vi "WPI_MotorControlSetOutput.vi"(8 "error in (no error)":errorcluster, 9 "options":u8, 10 "Output":dbl, 11 "MotorControlDevRef":T1={"DeviceStatus"={"status"=FALSE, "code"=0, "source"=""}, "Type"=enum."PWM", "PWM"={"PWM Channel"=enum."Invalid", "DeadBand"={"Name"="", "maxPositivePwm"=0, "minPositivePwm"=0, "centerPwm"=0, "maxNegativePwm"=0, "minNegativePwm"=0, "angularRange"=0}}, "CAN"={"Device Number"=0, "SetOutput VI Ref"=variant(refnum<vi> refnum), "GetOutput VI Ref"=variant(refnum<vi> refnum), "Enable VI Ref"=variant(refnum<vi> refnum), "Disable VI Ref"=variant(refnum<vi> refnum), "Data"=variant}, "Invert"=FALSE, "DIO PWM"={"PWM \"Enable\" Channel"=enum."Invalid", "DIOChannel"=enum."Invalid", "PWM Rate"=0.0}}) -> (0 "error out":errorcluster, 2 "Motor Output":dbl, 3 "MotorControlDevRef":T1={"DeviceStatus"={"status"=FALSE, "code"=0, "source"=""}, "Type"=enum."PWM", "PWM"={"PWM Channel"=enum."Invalid", "DeadBand"={"Name"="", "maxPositivePwm"=0, "minPositivePwm"=0, "centerPwm"=0, "maxNegativePwm"=0, "minNegativePwm"=0, "angularRange"=0}}, "CAN"={"Device Number"=0, "SetOutput VI Ref"=variant(refnum<vi> refnum), "GetOutput VI Ref"=variant(refnum<vi> refnum), "Enable VI Ref"=variant(refnum<vi> refnum), "Disable VI Ref"=variant(refnum<vi> refnum), "Data"=variant}, "Invert"=FALSE, "DIO PWM"={"PWM \"Enable\" Channel"=enum."Invalid", "DIOChannel"=enum."Invalid", "PWM Rate"=0.0}})   [LabVIEW 2025]
doc: "Specifies the output value or set-point for the motor controller.\n\nIf you use a motor controller connected to PWM, the scaled value can range from -1.0 to 1.0.\n\nIf you use a CAN Jaguar, the scale and the units depend on the mode the Jaguar is in. In <B>Percent VBus</B> mode, the range is the same as the PWM interface. In <B>Voltage</B>, <B>Current</B>, <B>Speed</B>, and <B>Position</B> modes, the <B>Output</B> is specified in engineering units (Volts, Amps, Rotations/Minute, and Rotations respectively).\n\nIf you use a CAN Talon SRX, the scale and the units depend on the mode the Talon SRXis in. In <B>Percent VBus</B> mode, the range is the same as the PWM interface. In <B>Speed</B>, and <B>Position</B> modes, the <B>Output</B> is specified in raw sensor units (ticks and ticks / 100 ms respectively).\n\nThe scale and units for other CAN motor controllers may be defined by the manufacturer.\n\nThis software is licensed. Open the labview\\readme\\WPI Robotics Library Open Source License.txt file for more information."
uses:
  <vilib>/Rock Robotics/WPI/MotorControl/WPI_MotorControlDeviceRef.ctl
  <vilib>/Rock Robotics/WPI/MotorControl/WPI_MotorControlType.ctl
  <vilib>/Rock Robotics/SystemInterfaces/DIO/FPGA_DIOPWMChannel.ctl
  <vilib>/Rock Robotics/WPI/PWM/WPI_PWMDeadband.ctl
  <vilib>/Rock Robotics/SystemInterfaces/DIO/FPGA_DIOChannel.ctl
  <vilib>/Rock Robotics/WPI/PWM/WPI_PWMChannelCacheOp.ctl
  <vilib>/Rock Robotics/WPI/MotorControl/WPI_MotorControlSafetyCheck.vi
  <instrlib>/DC Motor Controller/HAIOL/DC Motor Controller.lvclass
  <vilib>/Rock Robotics/WPI/MotorControl/WPI_MotorControlSetOutputRefType.ctl
  <vilib>/Rock Robotics/WPI/DigitalOutput/WPI_DigitalOutputDevRef.ctl
  <vilib>/Rock Robotics/WPI/Simulation/Protocol/Devices/PWM/PWM Update Ops.ctl
panel:
  in  "Sync Group":u8
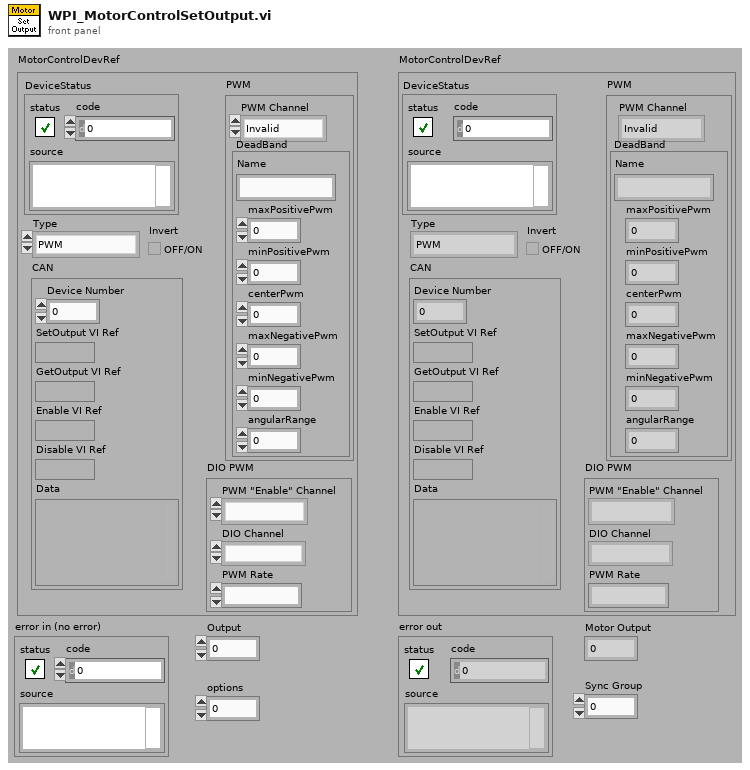
[diagram p1: front panel]
types:
  T1 = typedef "WPI_MotorControlDeviceRef.ctl" = cluster{"DeviceStatus":errorcluster, "Type":T2, "PWM":cluster{"PWM Channel":T3, "DeadBand":T4}, "CAN":cluster{"Device Number":u8, "SetOutput VI Ref":variant, "GetOutput VI Ref":variant, "Enable VI Ref":variant, "Disable VI Ref":variant, "Data":variant}, "Invert":bool, "DIO PWM":cluster{"PWM \"Enable\" Channel":T3, "DIOChannel":T5, "PWM Rate":dbl}}
  T2 = typedef "WPI_MotorControlType.ctl" = enum16{"PWM", "CAN", "DIO PWM"}
  T3 = typedef "FPGA_DIOPWMChannel.ctl" = enum8{"PWM 0", "PWM 1", "PWM 2", "PWM 3", "PWM 4", "PWM 5", "PWM 6", "PWM 7", "PWM 8", "PWM 9", "PWM MXP 0", "PWM MXP 1", "PWM MXP 2", "PWM MXP 3", "PWM MXP 4", "PWM MXP 5", "PWM MXP 6", "PWM MXP 7", "PWM MXP 8", "PWM MXP 9", "Invalid"}
  T4 = typedef "WPI_PWMDeadband.ctl" = cluster{"Name":string, "maxPositivePwm":i32, "minPositivePwm":i32, "centerPwm":i32, "maxNegativePwm":i32, "minNegativePwm":i32, "angularRange":u16}
  T5 = typedef "FPGA_DIOChannel.ctl" = enum8{"DIO 0", "DIO 1", "DIO 2", "DIO 3", "DIO 4", "DIO 5", "DIO 6", "DIO 7", "DIO 8", "DIO 9", "DIO MXP 0", "DIO MXP 1", "DIO MXP 2", "DIO MXP 3", "DIO MXP 4", "DIO MXP 5", "DIO MXP 6", "DIO MXP 7", "DIO MXP 8", "DIO MXP 9", "DIO MXP 10", "DIO MXP 11", "DIO MXP 12", "DIO MXP 13", "DIO MXP 14", "DIO MXP 15", "SPI Port CS1", "SPI Port CS2", "SPI Port CS3", "SPI Port MISO", "SPI Port MOSI", "Invalid"}
  T6 = typedef "WPI_PWMChannelCacheOp.ctl" = enum16{"Acquire", "Release", "Status"}
  T7 = typedef "WPI_MotorControlSetOutputRefType.ctl" = refnum<vi>
  T8 = typedef "WPI_DigitalOutputDevRef.ctl" = cluster{"DIO Channel":T5, "DevStatus":errorcluster}
  T9 = typedef "PWM Update Ops.ctl" = enum16{"set init", "set speed", "set position", "set raw", "set  period_scale", "set zero_latch", "set angular range", "get", "delete", "JSON update", "set name", "transmit initial", "reset"}
  T10 = typedef "FPGA_DIODevRef.ctl" = cluster{"DevStatus":errorcluster}
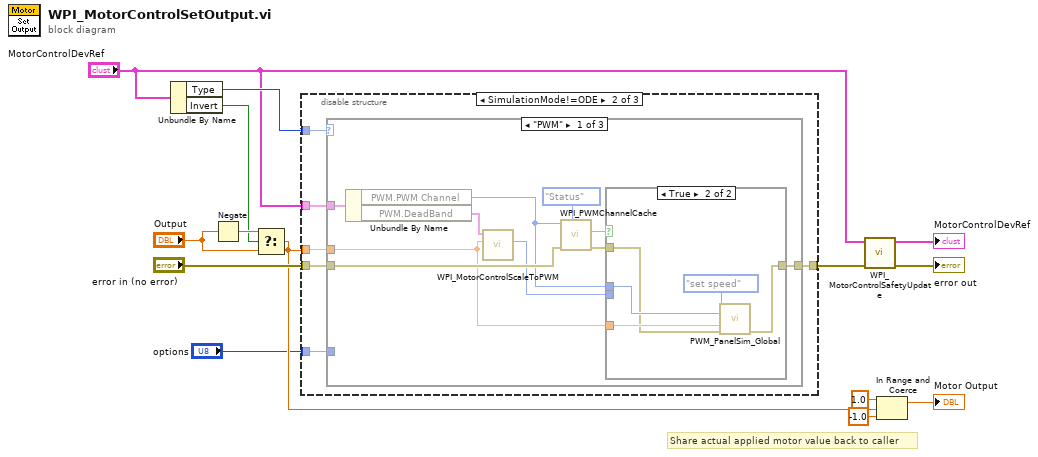
[diagram p0: block diagram]
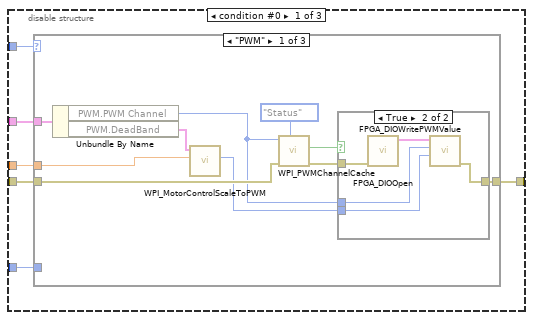
[diagram p2: hidden frame]
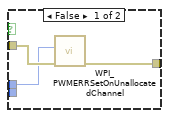
[diagram p3: hidden frame]
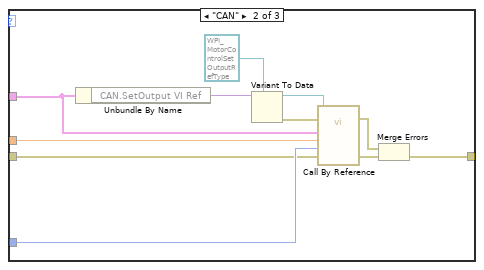
[diagram p4: hidden frame]
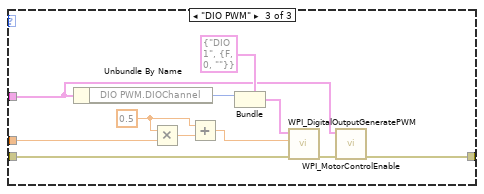
[diagram p5: hidden frame]
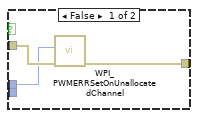
[diagram p6: hidden frame]
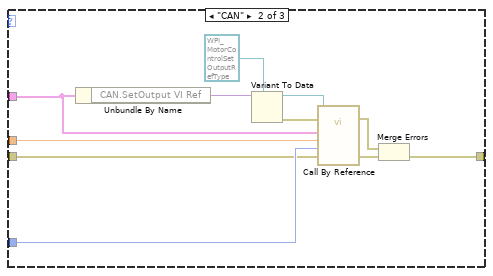
[diagram p7: hidden frame]
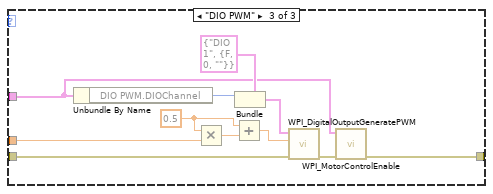
[diagram p8: hidden frame]
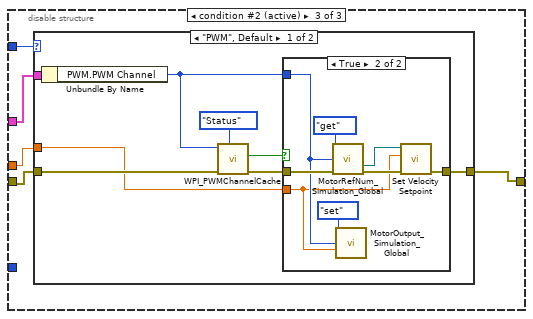
[diagram p9: hidden frame]
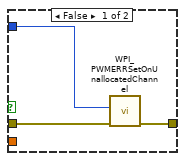
[diagram p10: hidden frame]
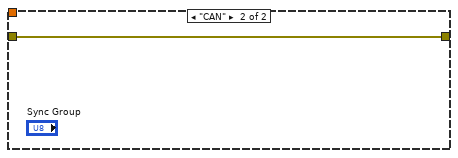
[diagram p11: hidden frame]
diagram:
  # "Share actual applied motor value back to caller"
  n1 = Unbundle By Name("MotorControlDevRef") -> ("Type"=w8:T2, "Invert"=w9:bool)
  n2 = Negate(x="Output") -> (-x=w10:dbl)
  n3 = Select(t=w10, s=w9, f="Output") -> (s? t:f=w3:dbl)
  n4 = disable-structure shown="SimulationMode!=ODE" {
    disable-tunnel: "error in (no error)" -> [w20 w66 w108]
    disable-tunnel: w8 -> [w19 w65 w111]
    disable-tunnel: [w18 w64 w107] -> w7
    disable-tunnel: "MotorControlDevRef" -> [w17 w63 w110]
    disable-tunnel: w3 -> [w16 w62 w109]
    disable-tunnel: "options" -> [w15 w61 _]
    frame condition #0 {
      n5 = case shown="\"PWM\"" w19 {
        tunnel: w20 -> [w26 w44 w53]
        tunnel: w16 -> [w30 w49 w57]
        tunnel: [w23 w41 w51] -> w18
        tunnel: w17 -> [w25 w45 w50]
        tunnel: w15 -> [_ w48 _]
        frame "PWM" {
          n6 = Unbundle By Name(w25) -> ("PWM.PWM Channel"=w22:T3, "PWM.DeadBand"=w21:T4)
          n7 = call <vilib>:"WPI_MotorControlScaleToPWM.vi"("Output (1,-1)"=w30, "DeadBand Info"=w21) -> ("Raw PWM Value"=w24:u16)  [unwired: 9 out]
          n8 = call <vilib>:"WPI_PWMChannelCache.vi"("Operation"=WPI_PWMChannelCacheOp."Status", "error in (no error)"=w26, "PWMChannel"=w22) -> ("error out"=w28:errorcluster, "Allocated?"=w29:bool)  [unwired: 2 in, 5 out]
          n9 = case shown="True" w29 {
            tunnel: w28 -> [w33 w37]
            tunnel: w22 -> [w31 w36]
            tunnel: [w32 w34] -> w23
            tunnel: w24 -> [_ w35]
            frame False {
              n10 = call <vilib>:"WPI_PWMERRSetOnUnallocatedChannel.vi"("error in (no error)"=w33, "PWM Channel"=w31) -> ("error out"=w32:errorcluster)  [unwired: 9 in]
            }
            frame True {
              n11 = call <vilib>:"FPGA_DIOOpen.vi"("error in (no error)"=w37) -> ("DIODeviceRef"=w38:T10)  [unwired: 1 in, 9 out]
              n12 = call <vilib>:"FPGA_DIOWritePWMValue.vi"("PWMValue"=w35, "PWMChannel"=w36, "DIODeviceRef In"=w38) -> ("error out"=w34:errorcluster)  [unwired: 2 in, 6 out]
            }
          }
        }
        frame "CAN" {
          n13 = Unbundle By Name(w45) -> ("CAN.SetOutput VI Ref"=w46:variant)
          n14 = Variant To Data(type=T7 refnum ("MotorControlSetOutput"), Variant=w46) -> (data=w47:T7, error out=w43:errorcluster)  [unwired: 1 in]
          n15 = call-by-ref "?"(reference=w47, error in=w43, 8:"error in (no error)"=w44, "options"=w48, "Output"=w49, "MotorControlDevRef"=w45) -> (error out=w40:errorcluster, 0:"error out"=w42:errorcluster)  [unwired: 5 in, 3 out]
          n16 = Merge Errors(w40, w42) -> (w41:errorcluster)
        }
        frame "DIO PWM" {
          w55 = 0.5 ("x")
          n17 = Unbundle By Name(w50) -> ("DIO PWM.DIOChannel"=w59:T5)
          n18 = Multiply(x=w55, y=w57) -> (x*y=w56:dbl)
          n19 = Add(x=w55, y=w56) -> (x+y=w54:dbl)
          n20 = Bundle(cluster=T8 {"DIO Channel"=enum."DIO 1", "DevStatus"={"status"=FALSE, "code"=0, "source"=""}} ("DigitalOutputDevRef"), "DIO Channel"=w59) -> (w58:T8)  [unwired: 1 in]
          n21 = call <vilib>:"WPI_DigitalOutputGeneratePWM.vi"("error in (no error)"=w53, "PWM Duty Cycle"=w54, "DigitalOutputDevRef"=w58) -> ("error out"=w52:errorcluster)  [unwired: 7 in, 1 out]
          n22 = call <vilib>:"WPI_MotorControlEnable.vi"("error in (no error)"=w52, "CAN MotorDevRef"=w50) -> ("error out"=w51:errorcluster)  [unwired: 8 in, 1 out]
        }
      }
    }
    frame condition #1 {
      n23 = case shown="\"PWM\"" w65 {
        tunnel: w66 -> [w73 w90 w99]
        tunnel: w62 -> [w67 w95 w103]
        tunnel: [w70 w87 w97] -> w64
        tunnel: w63 -> [w72 w91 w96]
        tunnel: w61 -> [_ w94 _]
        frame "PWM" {
          n24 = Unbundle By Name(w72) -> ("PWM.PWM Channel"=w69:T3, "PWM.DeadBand"=w68:T4)
          n25 = call <vilib>:"WPI_MotorControlScaleToPWM.vi"("Output (1,-1)"=w67, "DeadBand Info"=w68) -> ("Raw PWM Value"=w71:u16)  [unwired: 9 out]
          n26 = call <vilib>:"WPI_PWMChannelCache.vi"("Operation"=WPI_PWMChannelCacheOp."Status", "error in (no error)"=w73, "PWMChannel"=w69) -> ("error out"=w75:errorcluster, "Allocated?"=w76:bool)  [unwired: 2 in, 5 out]
          n27 = case shown="True" w76 {
            tunnel: w75 -> [w79 w80]
            tunnel: w69 -> [w77 w81]
            tunnel: [w78 w84] -> w70
            tunnel: w71 -> [_ _]
            tunnel: w67 -> [_ w82]
            frame False {
              n28 = call <vilib>:"WPI_PWMERRSetOnUnallocatedChannel.vi"("error in (no error)"=w79, "PWM Channel"=w77) -> ("error out"=w78:errorcluster)  [unwired: 9 in]
            }
            frame True {
              n29 = call <vilib>:"PWM_PanelSim_Global.vi"("menu"=PWM_Update_Ops."set speed", "PWMChannel"=w81, "Numeric Value"=w82, "error in (no error)"=w80) -> ("error out"=w84:errorcluster)  [unwired: 10 in, 1 out]
            }
          }
        }
        frame "CAN" {
          n30 = Unbundle By Name(w91) -> ("CAN.SetOutput VI Ref"=w92:variant)
          n31 = Variant To Data(type=T7 refnum ("MotorControlSetOutput"), Variant=w92) -> (data=w93:T7, error out=w89:errorcluster)  [unwired: 1 in]
          n32 = call-by-ref "?"(reference=w93, error in=w89, 8:"error in (no error)"=w90, "options"=w94, "Output"=w95, "MotorControlDevRef"=w91) -> (error out=w86:errorcluster, 0:"error out"=w88:errorcluster)  [unwired: 5 in, 3 out]
          n33 = Merge Errors(w86, w88) -> (w87:errorcluster)
        }
        frame "DIO PWM" {
          w101 = 0.5 ("x")
          n34 = Unbundle By Name(w96) -> ("DIO PWM.DIOChannel"=w105:T5)
          n35 = Multiply(x=w101, y=w103) -> (x*y=w102:dbl)
          n36 = Add(x=w101, y=w102) -> (x+y=w100:dbl)
          n37 = Bundle(cluster=T8 {"DIO Channel"=enum."DIO 1", "DevStatus"={"status"=FALSE, "code"=0, "source"=""}} ("DigitalOutputDevRef"), "DIO Channel"=w105) -> (w104:T8)  [unwired: 1 in]
          n38 = call <vilib>:"WPI_DigitalOutputGeneratePWM.vi"("error in (no error)"=w99, "PWM Duty Cycle"=w100, "DigitalOutputDevRef"=w104) -> ("error out"=w98:errorcluster)  [unwired: 7 in, 1 out]
          n39 = call <vilib>:"WPI_MotorControlEnable.vi"("error in (no error)"=w98, "CAN MotorDevRef"=w96) -> ("error out"=w97:errorcluster)  [unwired: 8 in, 1 out]
        }
      }
    }
    frame condition #2 (active) {
      n40 = case shown="\"PWM\", Default" w111 {
        tunnel: w108 -> [w115 w131]
        tunnel: w109 -> [w112 _]
        tunnel: [w114 w131] -> w107
        tunnel: w110 -> [w119 _]
        frame "PWM", Default {
          n41 = Unbundle By Name(w119) -> ("PWM.PWM Channel"=w113:T3)
          n42 = call <vilib>:"WPI_PWMChannelCache.vi"("Operation"=WPI_PWMChannelCacheOp."Status", "error in (no error)"=w115, "PWMChannel"=w113) -> ("error out"=w117:errorcluster, "Allocated?"=w116:bool)  [unwired: 2 in, 5 out]
          n43 = case shown="True" w116 {
            tunnel: w117 -> [w122 w129]
            tunnel: [w121 w126] -> w114
            tunnel: w113 -> [w120 w124]
            tunnel: w112 -> [_ w123]
            frame False {
              n44 = call <vilib>:"WPI_PWMERRSetOnUnallocatedChannel.vi"("error in (no error)"=w122, "PWM Channel"=w120) -> ("error out"=w121:errorcluster)  [unwired: 9 in]
            }
            frame True {
              n45 = call <vilib>:"MotorRefNum_Simulation_Global.vi"("menu"=enum16{"set", "get", "delete"}."get", "PWM Channel"=w124, "error in (no error)"=w129) -> ("DC Motor Controller Get"=w127:refnum<class "DC Motor Controller.lvclass">, "error out"=w128:errorcluster)  [unwired: 11 in]
              n46 = call <vilib>:"MotorOutput_Simulation_Global.vi"("menu"=enum16{"set", "get", "delete"}."set", "PWM Channel"=w124, "Output Set"=w123) -> ()  [unwired: 11 in, 2 out]
              n47 = call-dynamic "Set Velocity Setpoint.vi"("error in (no error)"=w128, "CCW Velocity (0 rad/s)"=w123, "DC Motor Controller in"=w127) -> ("error out"=w126:errorcluster)  [unwired: 7 in, 1 out]
            }
          }
        }
        frame "CAN" {
        }
      }
    }
  }
  n48 = call <vilib>:"WPI_MotorControlSafetyUpdate.vi"("error in (no error)"=w7, "MotorControlDevRef"="MotorControlDevRef") -> ("error out"=→"error out":errorcluster, "MotorControlDevRef"=→"MotorControlDevRef":T1)  [unwired: 8 out]
  n49 = In Range and Coerce(upper limit=1.0, x=w3, lower limit=-1.0) -> (coerced(x)=→"Motor Output":dbl)  [unwired: 1 out]
